vi "rs3 get device count2.vi"(8 "error in":errorcluster, 11 "device":u32) -> (0 "error out":errorcluster, 1 "device list":u32, 2 "device count":i32, 3 "error":u64)   [LabVIEW 2023]
doc: "Determine number of connected DEVICES."
panel:
  # "RS3 Get Device Count2"
  # "(C) Intel Corp.,  AGJ"
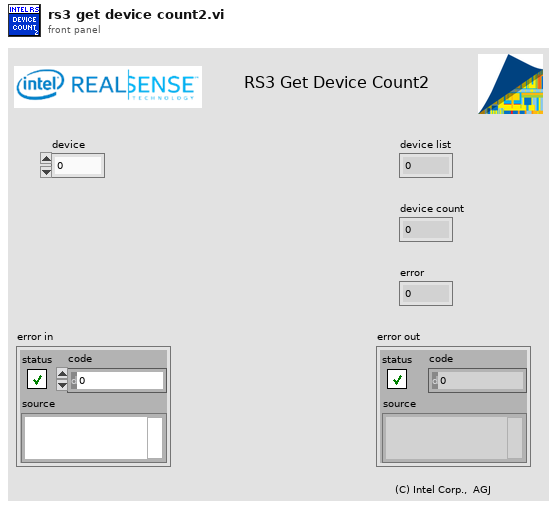
[diagram p1: front panel]
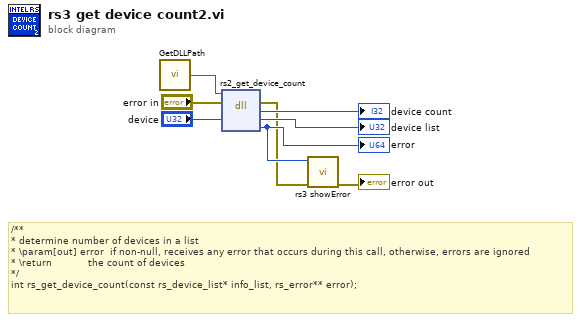
[diagram p0: block diagram]
diagram:
  # "/**\n* determine number of devices in a list\n* \\param[out] error  if non-null, receives any error that occurs during this call, otherwise, errors are ignored\n* \\return            the count of devices\n*/\nint rs_get_device_count(const rs_device_list* info_list, rs_error** error);"
  n1 = call "GetDLLPath.vi"() -> ("DLL Path"=w1:path)
  n2 = dll-call lib="C:/STEAMSyndicate/RealSenseWrappers/VI Wrappers (add ons) Public/RealSense/realsense2.dll" fn="rs2_get_device_count"(path in=w1, error in="error in", "rscontext"="device") -> (error out=w3:errorcluster, "device count"=→"device count":i32, "rscontext"=→"device list":u64, "error"=w4:u64)  [unwired: 2 in, 1 out]
  "error" <- w4
  n3 = call "rs3 showError.vi"("error in (no error)"=w3, "error"=w4) -> ("error out"=→"error out":errorcluster)  [unwired: 5 in, 4 out]
